vi "X_2.083_StateMachine.vi"() -> ()   [LabVIEW 2022 SP3]
uses:
  States.ctl
  ServiceType.ctl
panel:
  in  "Fail servicing customer":bool
  in  "Out of service 2":enum32{"Cancel", "Insert card", "Wait"}(radio)=enum."Wait"
  in  "Idle":T1(radio)=enum."Wait"
  in  "full service? 2":T2
  in  "Out of service":enum32{"Shutdown", "Service", "Wait"}(radio)=enum."Wait"
  in  "full service?":T2
  out "Enum":T3=enum."OutOfService"
  in  "Turn On":bool
  in  "stop":bool
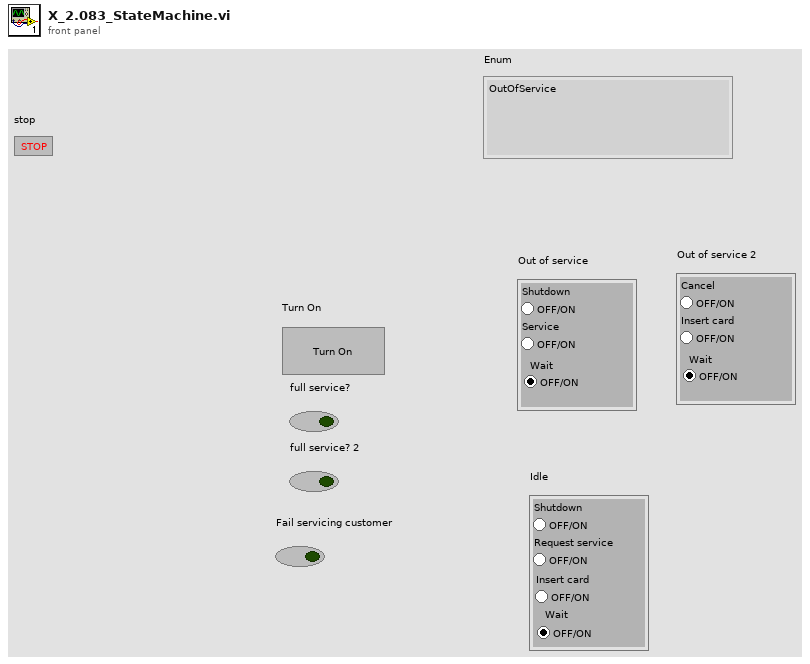
[diagram p1: front panel]
types:
  T1 = enum32{"Shutdown", "Request service", "Wait", "Insert card"}
  T2 = typedef "ServiceType.ctl" = bool
  T3 = typedef "States.ctl" = enum16{"Off", "Idle", "SelfTest", "Maintinance", "OutOfService", "ServicingCostummer"}
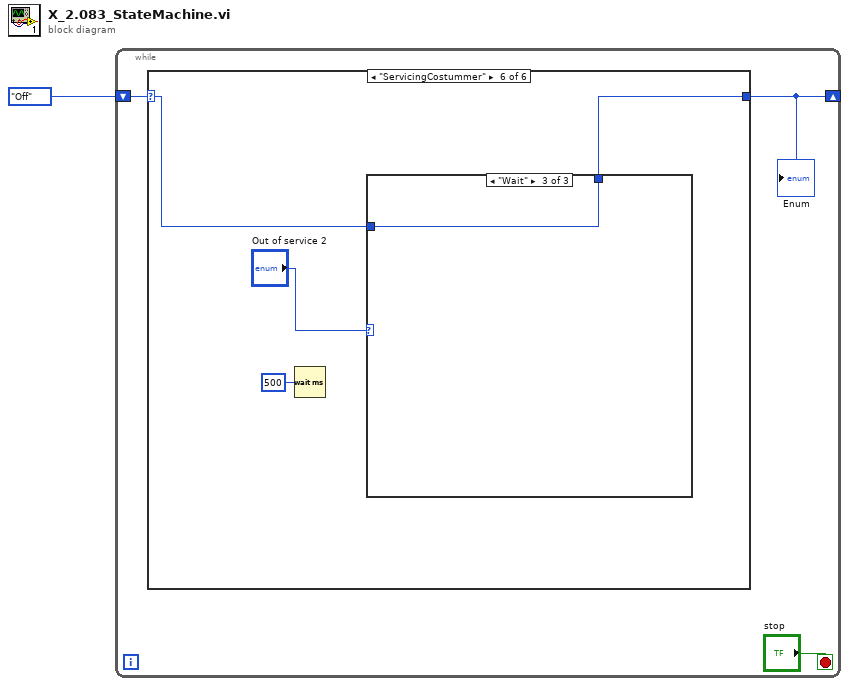
[diagram p0: block diagram]
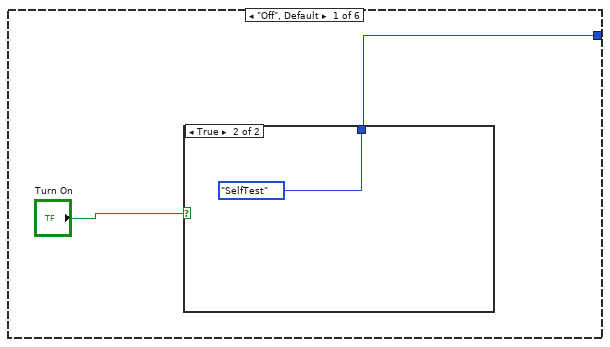
[diagram p2: hidden frame]
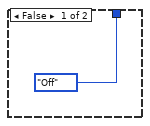
[diagram p3: hidden frame]
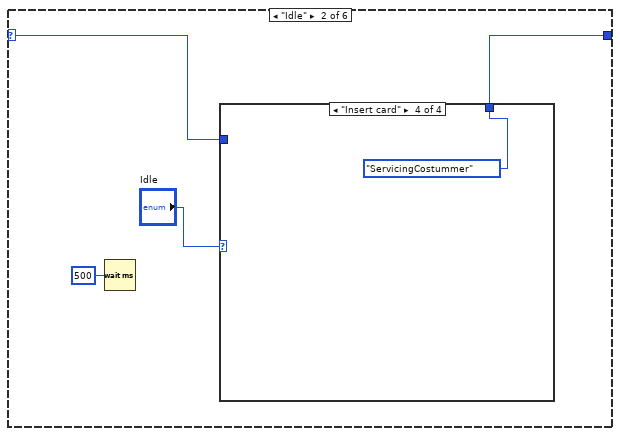
[diagram p4: hidden frame]
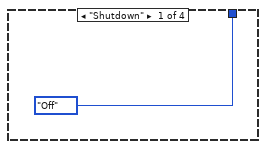
[diagram p5: hidden frame]
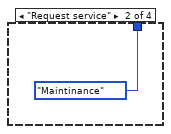
[diagram p6: hidden frame]
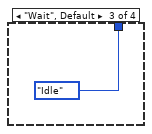
[diagram p7: hidden frame]
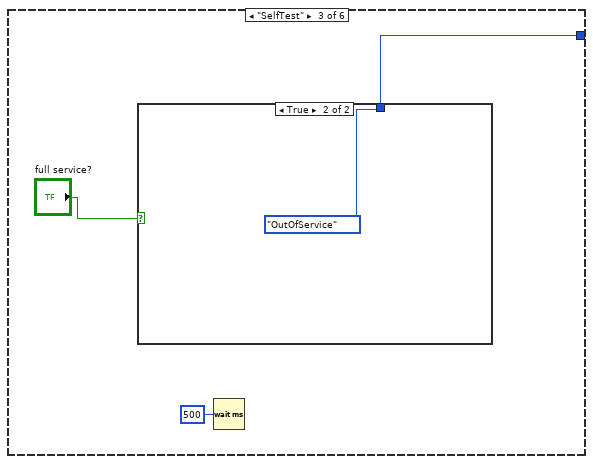
[diagram p8: hidden frame]
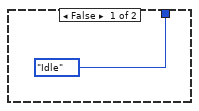
[diagram p9: hidden frame]
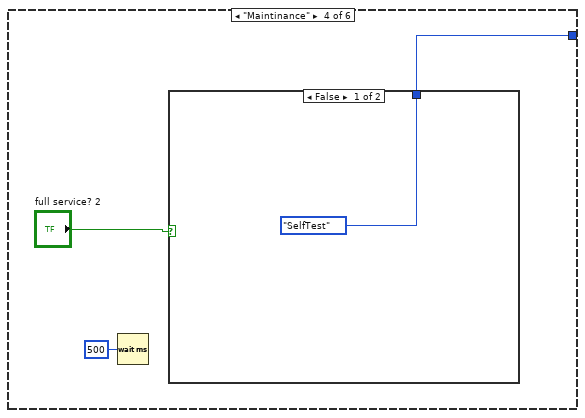
[diagram p10: hidden frame]
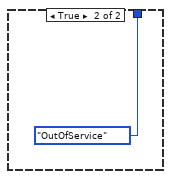
[diagram p11: hidden frame]
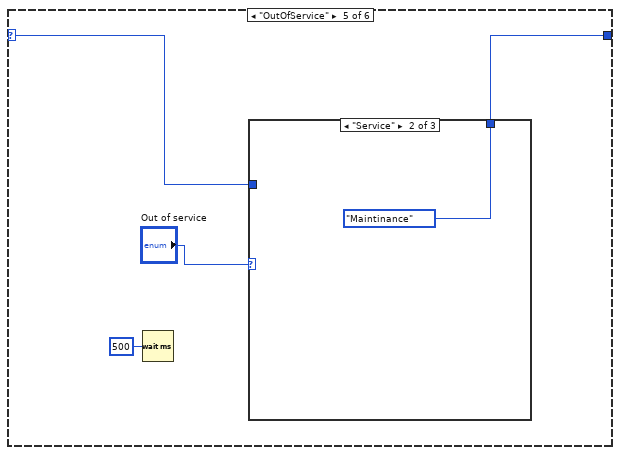
[diagram p12: hidden frame]
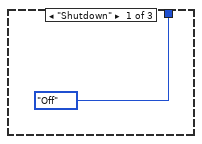
[diagram p13: hidden frame]
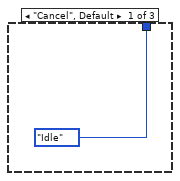
[diagram p15: hidden frame]
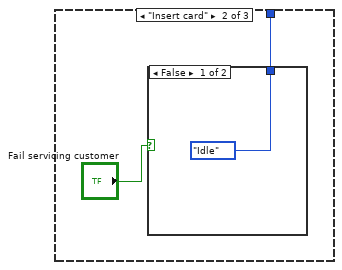
[diagram p16: hidden frame]
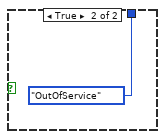
[diagram p17: hidden frame]
diagram:
  n1 = while {
    shift-right: [w2] -> _
    shift-left: States."Off" -> [w4]
    stop <- "stop" stop-if-true
    n2 = case shown="\"ServicingCostummer\"" w4 {
      selector: w4 -> [_ w10 _ _ w29 w35]
      tunnel: [w5 w9 w17 w22 w28 w36] -> w2
      frame "Off", Default {
        n3 = case shown="True" "Turn On" {
          tunnel: [States."Off" States."SelfTest"] -> w5
          frame False {
          }
          frame True {
          }
        }
      }
      frame "Idle" {
        n4 = Wait (ms)(milliseconds to wait=u32 500) -> ()  [unwired: 1 out]
        n5 = case shown="\"Insert card\"" "Idle" {
          tunnel: w10 -> [_ _ _ _]
          tunnel: [States."Off" States."Maintinance" States."Idle" States."ServicingCostummer"] -> w9
          frame "Shutdown" {
          }
          frame "Request service" {
          }
          frame "Wait", Default {
          }
          frame "Insert card" {
          }
        }
      }
      frame "SelfTest" {
        n6 = case shown="True" "full service?" {
          tunnel: [States."Idle" States."OutOfService"] -> w17
          frame False {
          }
          frame True {
          }
        }
        n7 = Wait (ms)(milliseconds to wait=u32 500) -> ()  [unwired: 1 out]
      }
      frame "Maintinance" {
        n8 = Wait (ms)(milliseconds to wait=u32 500) -> ()  [unwired: 1 out]
        n9 = case shown="False" "full service? 2" {
          tunnel: [States."SelfTest" States."OutOfService"] -> w22
          frame False {
          }
          frame True {
          }
        }
      }
      frame "OutOfService" {
        n10 = Wait (ms)(milliseconds to wait=u32 500) -> ()  [unwired: 1 out]
        n11 = case shown="\"Service\"" "Out of service" {
          tunnel: w29 -> [_ _ w33]
          tunnel: [States."Off" States."Maintinance" w33] -> w28
          frame "Shutdown" {
          }
          frame "Service" {
          }
          frame "Wait", Default {
          }
        }
      }
      frame "ServicingCostummer" {
        n12 = Wait (ms)(milliseconds to wait=u32 500) -> ()  [unwired: 1 out]
        n13 = case shown="\"Wait\"" "Out of service 2" {
          tunnel: [States."Idle" w39 w43] -> w36
          tunnel: w35 -> [_ _ w43]
          frame "Cancel", Default {
          }
          frame "Insert card" {
            n14 = case shown="False" "Fail servicing customer" {
              tunnel: [States."Idle" States."OutOfService"] -> w39
              frame False {
              }
              frame True {
              }
            }
          }
          frame "Wait" {
          }
        }
      }
    }
    "Enum" <- w2
  }
